vi "CreatePattern.vi"(4 "Color Box":u32=16724224, 5 "Pattern Type":T2 items=["Fringe Pattern (V)", "Fringe Pattern (H)", "Central Line (V)", "Central Line (H)", "Central Cross", "background-color"], 6 "Shift":dbl, 7 "Intensity":T1, 8 "Value":dbl=255.0, 9 "Pitch":dbl=20.0, 10 "Y":dbl[][](array[numeric]), 11 "X":dbl[][](array[numeric])) -> (2 "Real Matrix":T1, 3 "Refnum out":T3)   [LabVIEW 2015]
uses:
  <vilib>/vision/Image Controls.llb/IMAQ Image.ctl
  <vilib>/Analysis/Matrix/Datatypes/RealMatrix.ctl
  <vilib>/Analysis/Matrix/Numeric/Multiply/Multiply - RM,R.vi
  <vilib>/Analysis/Matrix/NI_Matrix.lvlib
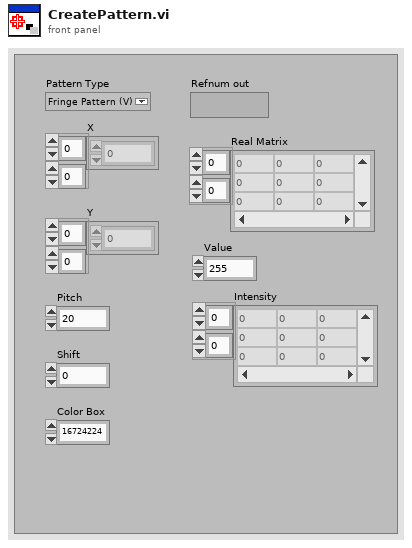
[diagram p1: front panel]
types:
  T1 = typedef "NI_Matrix.lvlib/RealMatrix.ctl" = dbl[][]
  T2 = typedef "Image Type" = u32
  T3 = typedef "IMAQ Image.ctl" = refnum<image>
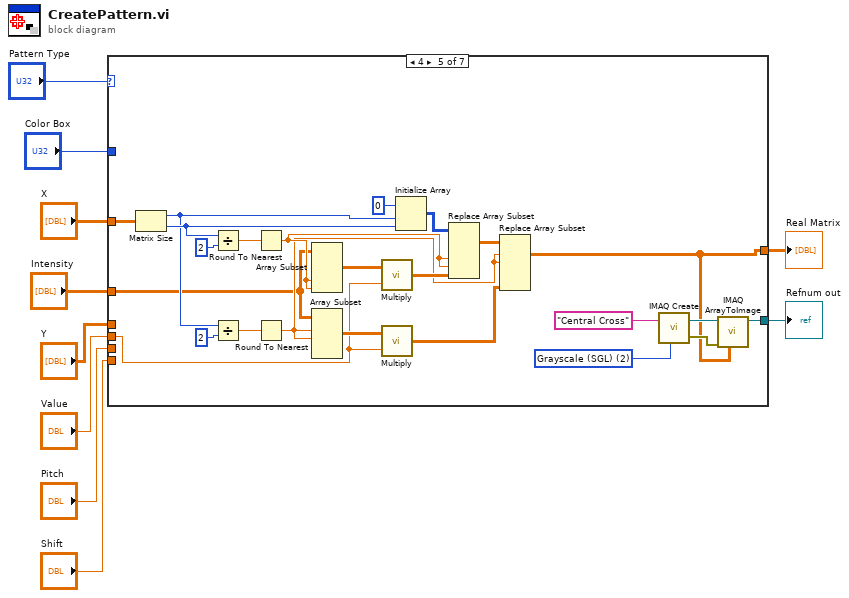
[diagram p0: block diagram]
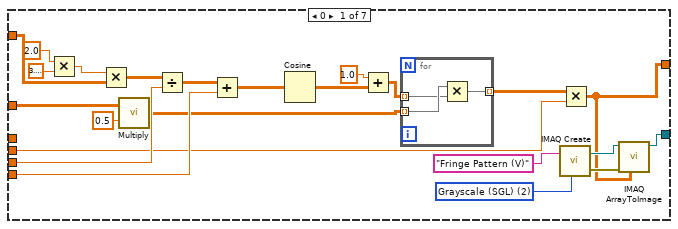
[diagram p2: hidden frame]
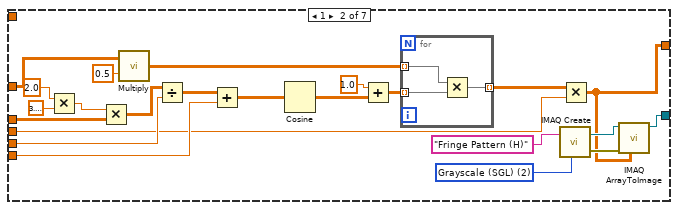
[diagram p3: hidden frame]
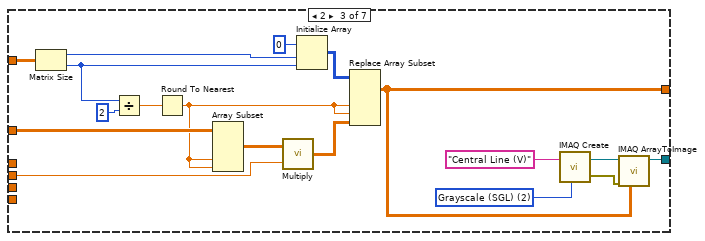
[diagram p4: hidden frame]
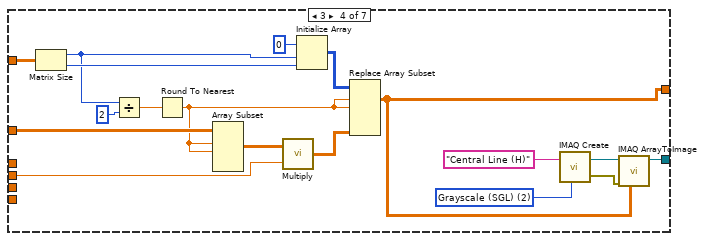
[diagram p5: hidden frame]
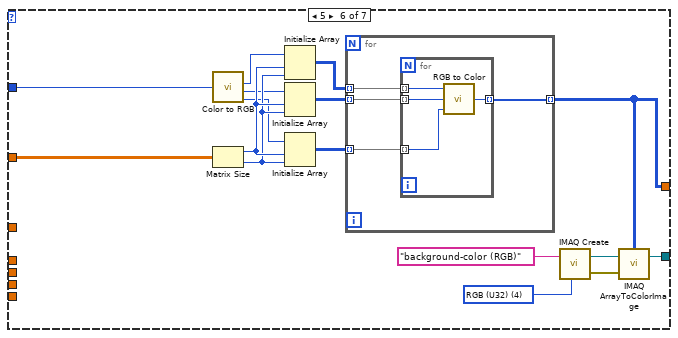
[diagram p6: hidden frame]
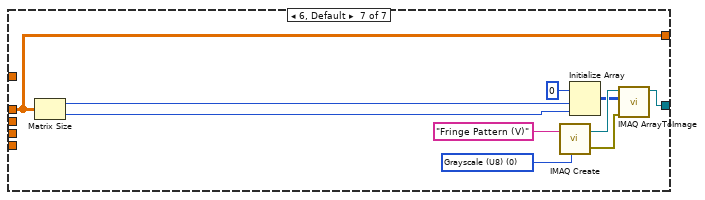
[diagram p7: hidden frame]
diagram:
  n1 = case shown="4" "Pattern Type" {
    tunnel: "X" -> [w17 _ w79 w90 w109 w138 _]
    tunnel: "Pitch" -> [w24 w42 _ _ _ _ _]
    tunnel: "Intensity" -> [w18 w43 w68 w86 w100 _ _]
    tunnel: "Shift" -> [w22 w41 _ _ _ _ _]
    tunnel: "Y" -> [_ w40 _ _ _ _ w153]
    tunnel: "Color Box" -> [_ _ _ _ _ w135 _]
    tunnel: [w21 w39 w63 w81 w99 w126 w153] -> w9
    tunnel: [w20 w38 w69 w87 w108 w125 w147] -> w10
    tunnel: "Value" -> [w19 w37 w65 w83 w102 _ _]
    frame 0 {
      w26 = T2 2 items=["Grayscale (U8)", "Grayscale (I16)", "Grayscale (SGL)", "Complex (CSG)", "RGB (U32)", "HSL (U32)", "RGB (U64)"] ("Image Type")
      n2 = Multiply(x=2.0, y=3.141592653589793) -> (x*y=w29:dbl)
      n3 = Multiply(x=w29, y=w17) -> (x*y=w16:dbl[][])
      n4 = call-poly <vilib>:"Multiply.vi"("Real Scalar c"=0.5, "Real Matrix A"=w18) -> ("A * c"=w12:T1)
      n5 = Divide(x=w16, y=w24) -> (x/y=w15:dbl[][])
      n6 = Add(x=w15, y=w22) -> (x+y=w23:dbl[][])
      n7 = Cosine(x=w23) -> (cos(x)=w14:dbl[][])
      n8 = Add(x=1.0, y=w14) -> (x+y=w11:dbl[][])
      n9 = for {
        tunnel: [w36] -> w13 mode=indexing
        tunnel: w12 -> [w35] mode=indexing
        tunnel: w11 -> [w34] mode=indexing
        n10 = Multiply ("Multiply.vi")(x=w35, y=w34) -> (x*y=w36:dbl[])
      }
      n11 = call "IMAQ Create"("Image Name"="Fringe Pattern (V)", "Image Type"=w26) -> ("New Image"=w28:T3, "error out"=w25:errorcluster)  [unwired: 3 in]
      n12 = Multiply ("Multiply.vi")(x=w13, y=w19) -> (x*y=w21:dbl[][])
      n13 = call "IMAQ ArrayToImage"("Image Pixels (Float)"=w21, "error in (no error)"=w25, "Image"=w28) -> ("Image Out"=w20:T3)  [unwired: 7 in, 1 out]
    }
    frame 1 {
      w47 = T2 2 items=["Grayscale (U8)", "Grayscale (I16)", "Grayscale (SGL)", "Complex (CSG)", "RGB (U32)", "HSL (U32)", "RGB (U64)"] ("Image Type")
      n14 = Multiply(x=2.0, y=3.141592653589793) -> (x*y=w53:dbl)
      n15 = Multiply(x=w53, y=w40) -> (x*y=w52:dbl[][])
      n16 = call-poly <vilib>:"Multiply.vi"("Real Scalar c"=0.5, "Real Matrix A"=w43) -> ("A * c"=w58:T1)
      n17 = Divide(x=w52, y=w42) -> (x/y=w45:dbl[][])
      n18 = Add(x=w45, y=w41) -> (x+y=w44:dbl[][])
      n19 = Cosine(x=w44) -> (cos(x)=w56:dbl[][])
      n20 = Add(x=1.0, y=w56) -> (x+y=w51:dbl[][])
      n21 = for {
        tunnel: w58 -> [w62] mode=indexing
        tunnel: w51 -> [w61] mode=indexing
        tunnel: [w60] -> w50 mode=indexing
        n22 = Multiply ("Multiply.vi")(x=w62, y=w61) -> (x*y=w60:dbl[])
      }
      n23 = call "IMAQ Create"("Image Name"="Fringe Pattern (H)", "Image Type"=w47) -> ("New Image"=w49:T3, "error out"=w46:errorcluster)  [unwired: 3 in]
      n24 = Multiply ("Multiply.vi")(x=w50, y=w37) -> (x*y=w39:dbl[][])
      n25 = call "IMAQ ArrayToImage"("Image Pixels (Float)"=w39, "error in (no error)"=w46, "Image"=w49) -> ("Image Out"=w38:T3)  [unwired: 7 in, 1 out]
    }
    frame 2 {
      w72 = T2 2 items=["Grayscale (U8)", "Grayscale (I16)", "Grayscale (SGL)", "Complex (CSG)", "RGB (U32)", "HSL (U32)", "RGB (U64)"] ("Image Type")
      n26 = Matrix Size(0:w79) -> (1:w78:i32, 2:w77:i32)
      n27 = Divide(x=w77, y=2) -> (x/y=w75:dbl)
      n28 = Round To Nearest(number=w75) -> (nearest integer value=w67:dbl)
      n29 = Array Subset(array=w68, index (col)=w67, length (col)=w67) -> (w66:T1)  [unwired: 2 in]
      n30 = call-poly <vilib>:"Multiply.vi"("Real Scalar c"=w65, "Real Matrix A"=w66) -> ("A * c"=w64:T1)
      n31 = Initialize Array(0, w78, w77) -> (w74:i32[][])
      n32 = Replace Array Subset(array=w74, new element=w64, index (dim 2)=w67, index (dim 3)=w67) -> (w63:T1)  [unwired: 2 in]
      n33 = call "IMAQ Create"("Image Name"="Central Line (V)", "Image Type"=w72) -> ("New Image"=w70:T3, "error out"=w71:errorcluster)  [unwired: 3 in]
      n34 = call "IMAQ ArrayToImage"("Image Pixels (Float)"=w63, "error in (no error)"=w71, "Image"=w70) -> ("Image Out"=w69:T3)  [unwired: 7 in, 1 out]
    }
    frame 3 {
      w92 = T2 2 items=["Grayscale (U8)", "Grayscale (I16)", "Grayscale (SGL)", "Complex (CSG)", "RGB (U32)", "HSL (U32)", "RGB (U64)"] ("Image Type")
      n35 = Matrix Size(0:w90) -> (1:w89:i32, 2:w97:i32)
      n36 = Divide(x=w89, y=2) -> (x/y=w95:dbl)
      n37 = Round To Nearest(number=w95) -> (nearest integer value=w85:dbl)
      n38 = Array Subset(array=w86, index (row)=w85, length (row)=w85) -> (w84:T1)  [unwired: 2 in]
      n39 = call-poly <vilib>:"Multiply.vi"("Real Scalar c"=w83, "Real Matrix A"=w84) -> ("A * c"=w82:T1)
      n40 = Initialize Array(0, w89, w97) -> (w94:i32[][])
      n41 = Replace Array Subset(array=w94, new element=w82, index (dim 0)=w85, index (dim 1)=w85) -> (w81:T1)  [unwired: 2 in]
      n42 = call "IMAQ Create"("Image Name"="Central Line (H)", "Image Type"=w92) -> ("New Image"=w88:T3, "error out"=w91:errorcluster)  [unwired: 3 in]
      n43 = call "IMAQ ArrayToImage"("Image Pixels (Float)"=w81, "error in (no error)"=w91, "Image"=w88) -> ("Image Out"=w87:T3)  [unwired: 7 in, 1 out]
    }
    frame 4 {
      w113 = T2 2 items=["Grayscale (U8)", "Grayscale (I16)", "Grayscale (SGL)", "Complex (CSG)", "RGB (U32)", "HSL (U32)", "RGB (U64)"] ("Image Type")
      n44 = Matrix Size(0:w109) -> (1:w115:i32, 2:w118:i32)
      n45 = Divide(x=w118, y=2) -> (x/y=w120:dbl)
      n46 = Divide(x=w115, y=2) -> (x/y=w116:dbl)
      n47 = Round To Nearest(number=w120) -> (nearest integer value=w107:dbl)
      n48 = Round To Nearest(number=w116) -> (nearest integer value=w104:dbl)
      n49 = Array Subset(array=w100, index (col)=w107, length (col)=w107) -> (w106:T1)  [unwired: 2 in]
      n50 = Array Subset(array=w100, index (row)=w104, length (row)=w104) -> (w103:T1)  [unwired: 2 in]
      n51 = call-poly <vilib>:"Multiply.vi"("Real Scalar c"=w102, "Real Matrix A"=w106) -> ("A * c"=w105:T1)
      n52 = call-poly <vilib>:"Multiply.vi"("Real Scalar c"=w102, "Real Matrix A"=w103) -> ("A * c"=w101:T1)
      n53 = Initialize Array(0, w115, w118) -> (w119:i32[][])
      n54 = Replace Array Subset(array=w119, new element=w105, index (dim 2)=w107, index (dim 3)=w107) -> (w111:T1)  [unwired: 2 in]
      n55 = Replace Array Subset(array=w111, new element=w101, index (dim 0)=w104, index (dim 1)=w104) -> (w99:T1)  [unwired: 2 in]
      n56 = call "IMAQ Create"("Image Name"="Central Cross", "Image Type"=w113) -> ("New Image"=w110:T3, "error out"=w112:errorcluster)  [unwired: 3 in]
      n57 = call "IMAQ ArrayToImage"("Image Pixels (Float)"=w99, "error in (no error)"=w112, "Image"=w110) -> ("Image Out"=w108:T3)  [unwired: 7 in, 1 out]
    }
    frame 5 {
      w127 = T2 4 items=["Grayscale (U8)", "Grayscale (I16)", "Grayscale (SGL)", "Complex (CSG)", "RGB (U32)", "HSL (U32)", "RGB (U64)"] ("Image Type")
      n58 = call <vilib>:"Color to RGB.vi"("Color"=w135) -> ("R"=w134:u8, "G"=w133:u8, "B"=w132:u8)  [unwired: 1 out]
      n59 = Matrix Size(0:w138) -> (1:w137:i32, 2:w136:i32)
      n60 = Initialize Array(w134, w137, w136) -> (w131:u8[][])
      n61 = Initialize Array(w133, w137, w136) -> (w130:u8[][])
      n62 = Initialize Array(w132, w137, w136) -> (w129:u8[][])
      n63 = for {
        tunnel: w131 -> [w142] mode=indexing
        tunnel: w130 -> [w141] mode=indexing
        tunnel: w129 -> [w140] mode=indexing
        tunnel: [w139] -> w126 mode=indexing
        n64 = for {
          tunnel: w142 -> [w146] mode=indexing
          tunnel: w141 -> [w145] mode=indexing
          tunnel: w140 -> [w144] mode=indexing
          tunnel: [w143] -> w139 mode=indexing
          n65 = call <vilib>:"RGB to Color.vi"("B"=w144, "G"=w145, "R"=w146) -> ("Color"=w143:u32)
        }
      }
      n66 = call "IMAQ Create"("Image Name"="background-color (RGB)", "Image Type"=w127) -> ("New Image"=w123:T3, "error out"=w124:errorcluster)  [unwired: 3 in]
      n67 = call "IMAQ ArrayToColorImage"("Image Pixels (U32)"=w126, "Image"=w123, "error in (no error)"=w124) -> ("Image Out"=w125:T3)  [unwired: 2 in, 1 out]
    }
    frame 6, Default {
      w150 = T2 0 items=["Grayscale (U8)", "Grayscale (I16)", "Grayscale (SGL)", "Complex (CSG)", "RGB (U32)", "HSL (U32)", "RGB (U64)"] ("Image Type")
      n68 = Matrix Size(0:w153) -> (1:w155:i32, 2:w154:i32)
      n69 = call "IMAQ Create"("Image Name"="Fringe Pattern (V)", "Image Type"=w150) -> ("New Image"=w152:T3, "error out"=w149:errorcluster)  [unwired: 3 in]
      n70 = Initialize Array(0, w155, w154) -> (w148:i32[][])
      n71 = call "IMAQ ArrayToImage"("error in (no error)"=w149, "Image Pixels (U8)"=w148, "Image"=w152) -> ("Image Out"=w147:T3)  [unwired: 7 in, 1 out]
    }
  }
  "Refnum out" <- w10
  "Real Matrix" <- w9
